vi "SUMMER SUNDAY BYTE[3].vi"() -> ()   [LabVIEW 2009]
uses:
  <vilib>/ULx/Create Channel.llb/ULx Create Channel (AI-Voltage-Basic).vi
  <vilib>/ULx/Read.llb/ULx Read (Analog DBL 1Chan 1Samp).vi
panel:
  out "POWER":bool
  out "data":dbl format="%_6g"
  out "xray":bool caption="BitValue"
  out "ENERGY LEVEL":dbl(knob) scale=0.0..15.0
  out "Beam Pot":dbl format="%_6g"
  out "READY 2":bool
  out "DUMP":bool
  out "POWER":bool
  out "?":bool
  out "?":bool
  out "?":bool
  out "?":bool
  out "?":bool
  out "?":bool
  out "?":bool
  out "?":bool
  out "?":bool
  out "?":bool
  out "OPEN":bool
  out "CLOSED":bool
  out "READY":bool
  out "FAULT":bool
  out "MAGNET FORCE":dbl(slide) scale=0.0..10.0
  out "READY":bool
  out "TEMPERATURE":dbl(slide) scale=0.0..100.0
  in  "stop":bool
  out "?":bool
  out "?":bool
  out "?":bool
  out "?":bool
  out "FAULT":bool
  out "POWER":bool
  out "FLOW IN GPM":dbl(knob) scale=0.0..15.0
  # "USERS LAB AREA"
  # "BEAM STATUS"
  # "ROOM"
  # "XRAY"
  # "PUMP STATION"
  # "MAGNET STATUS"
  # "ORBIT"
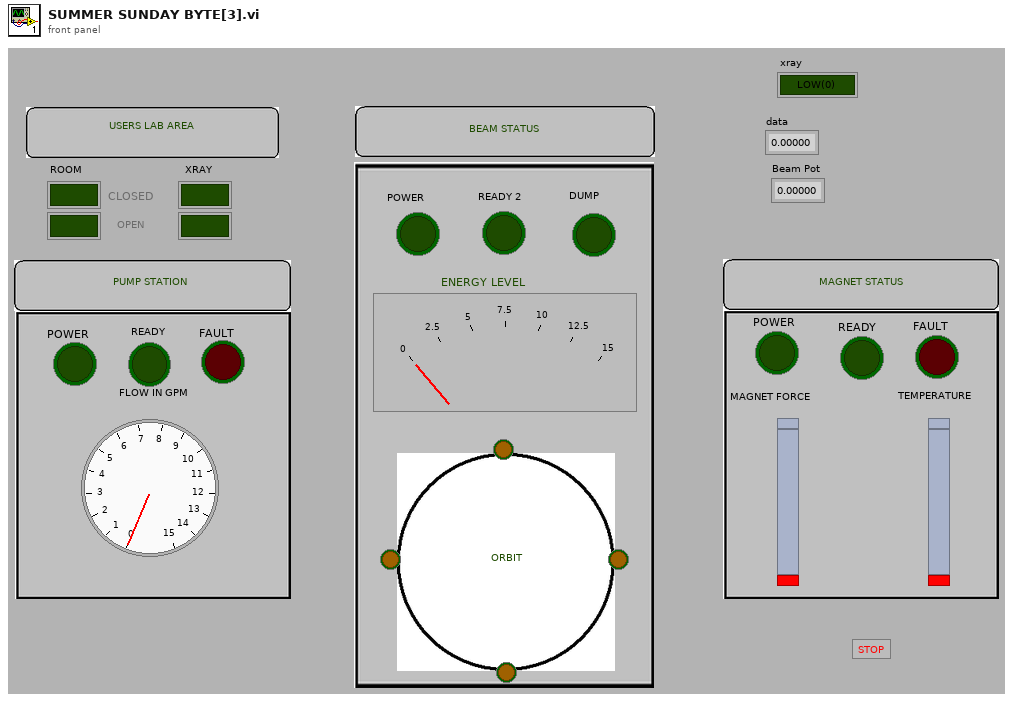
[diagram p1: front panel]
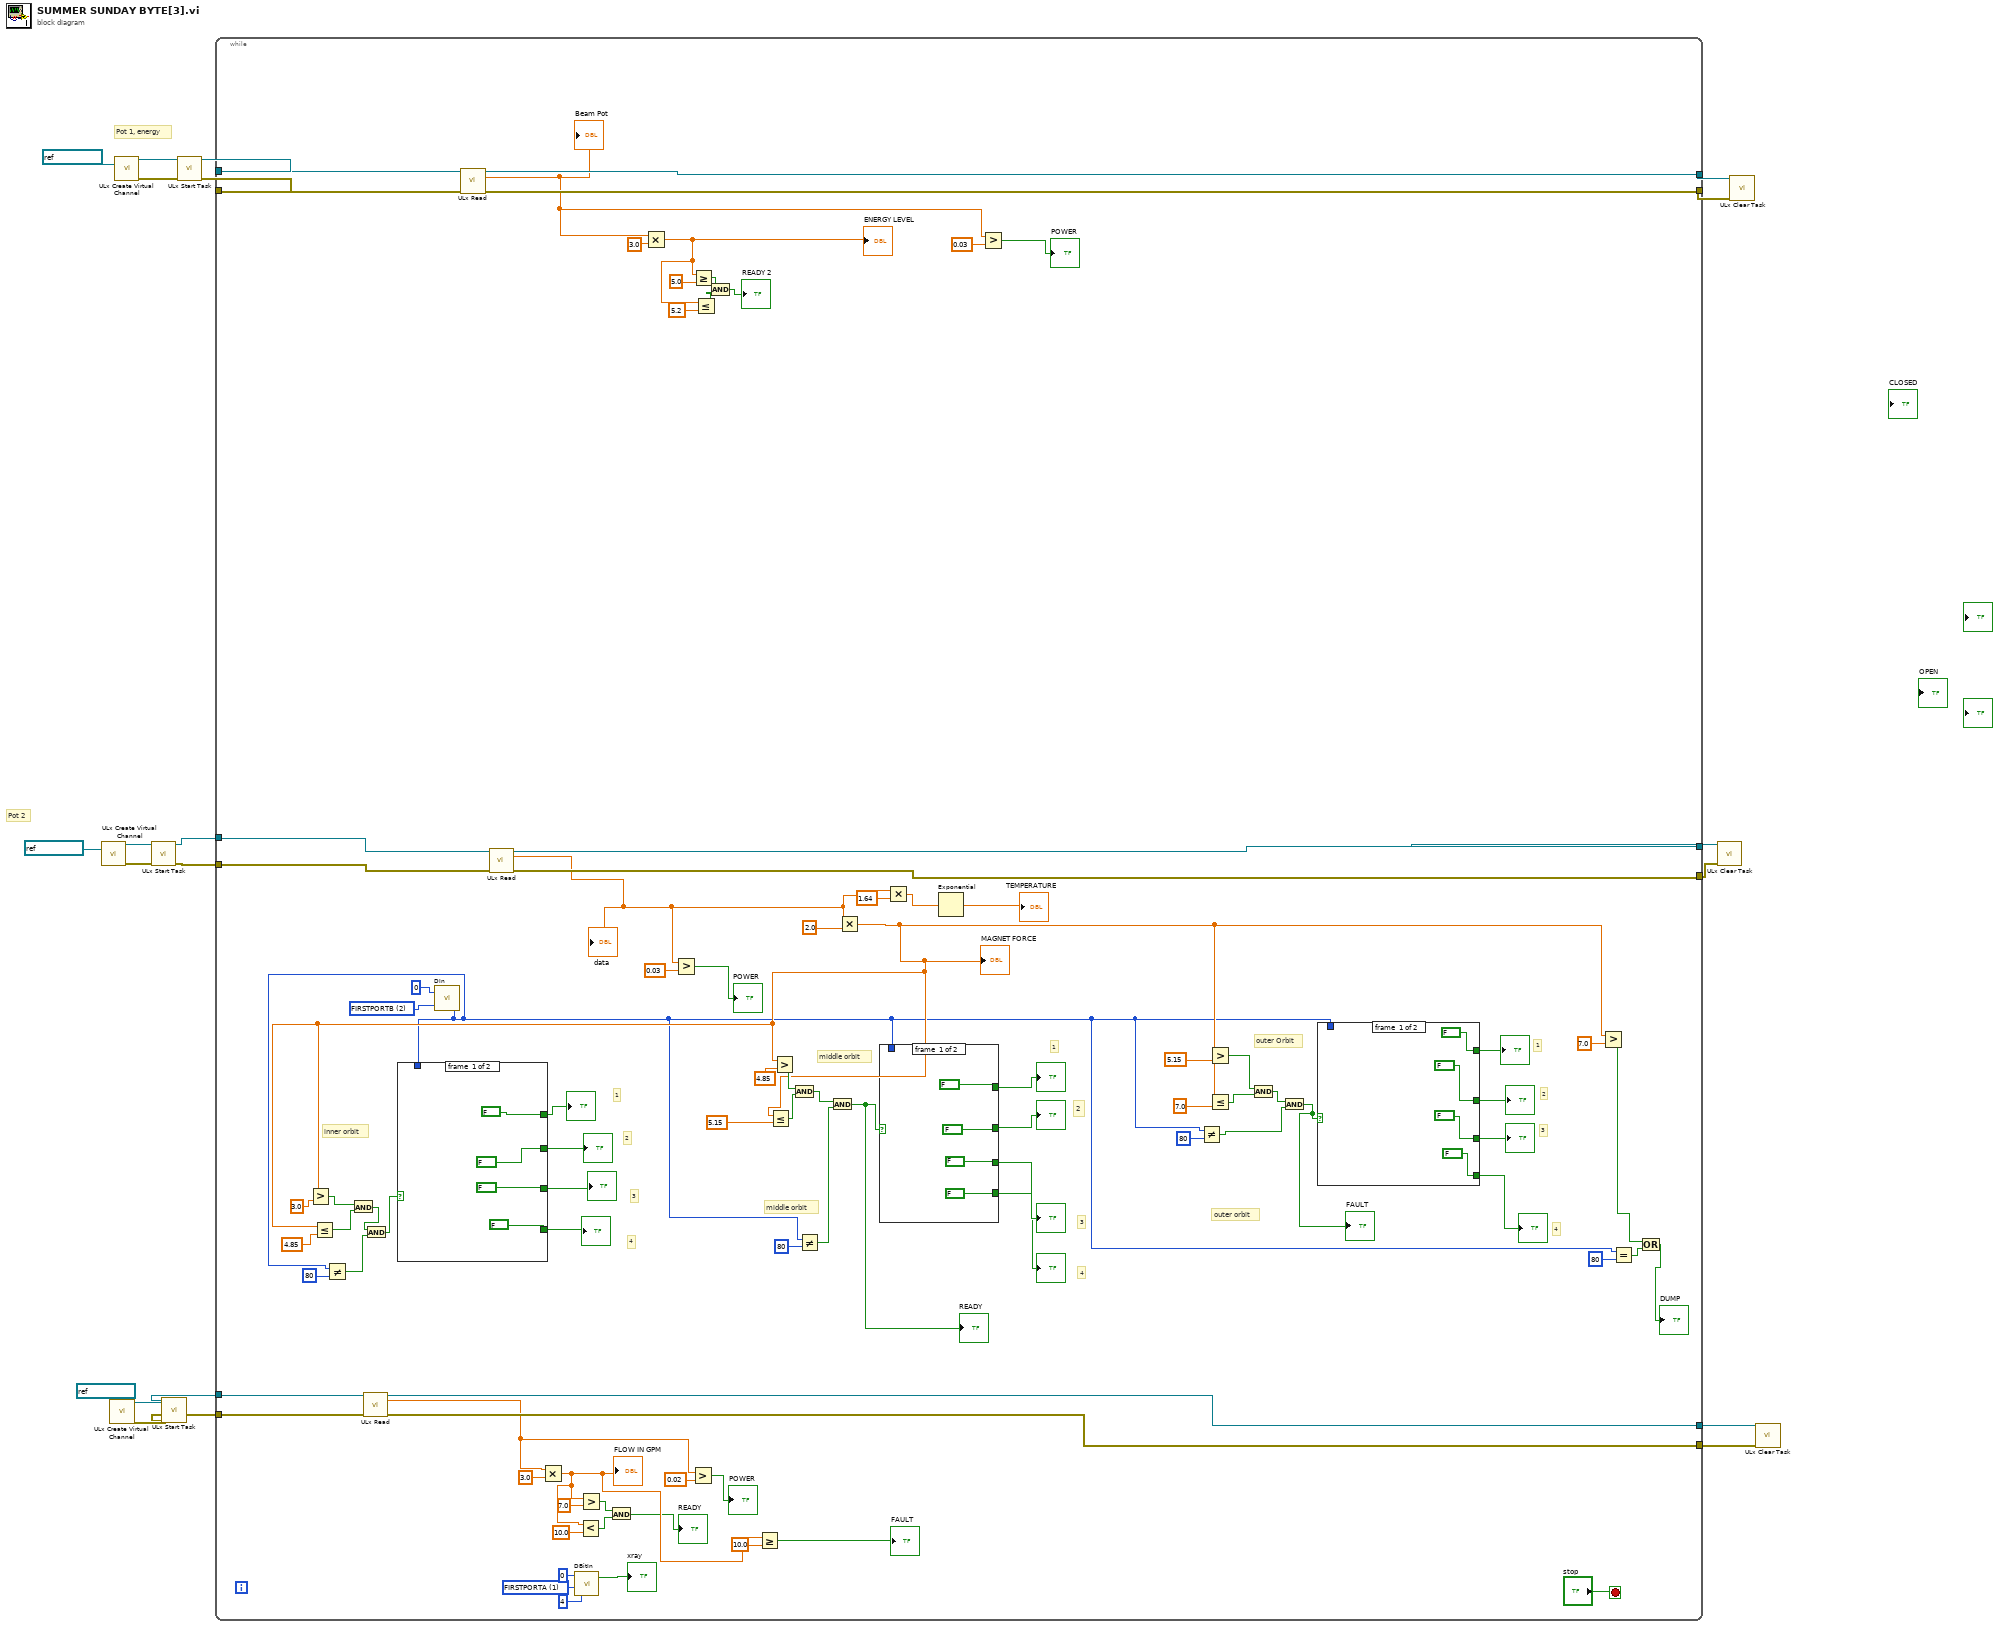
[diagram p0: block diagram]
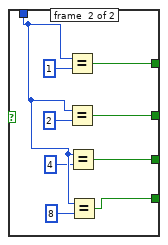
[diagram p2: hidden frame]
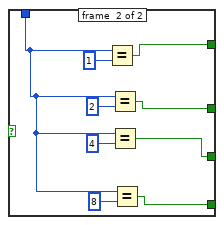
[diagram p3: hidden frame]
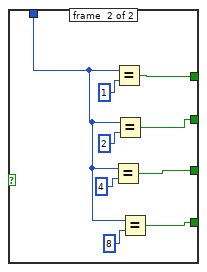
[diagram p4: hidden frame]
diagram:
  # "Pot 2"
  # "Pot 1, energy"
  n1 = call-poly <vilib>:"ULx Create Virtual Channel.vi"("physical channels"=refnum<k21> "Dev0/Ai1") -> ("task out"=w15:refnum<k24>, "error out"=w14:errorcluster)  [unwired: 13 in]
  n2 = call-poly <vilib>:"ULx Create Virtual Channel.vi"("physical channels"=refnum<k21> "Dev0/Ai2") -> ("task out"=w7:refnum<k24>, "error out"=w6:errorcluster)  [unwired: 13 in]
  n3 = call-poly <vilib>:"ULx Create Virtual Channel.vi"("physical channels"=refnum<k21> "Dev0/Ai0") -> ("task out"=w21:refnum<k24>, "error out"=w20:errorcluster)  [unwired: 13 in]
  n4 = call <vilib>:"ULx Start Task.vi"("task in"=w15, "error in"=w14) -> ("task out"=w13:refnum<k24>, "error out"=w12:errorcluster)  [unwired: 12 in]
  n5 = call <vilib>:"ULx Start Task.vi"("task in"=w7, "error in"=w6) -> ("task out"=w5:refnum<k24>, "error out"=w4:errorcluster)  [unwired: 12 in]
  n6 = call <vilib>:"ULx Start Task.vi"("task in"=w21, "error in"=w20) -> ("task out"=w19:refnum<k24>, "error out"=w18:errorcluster)  [unwired: 12 in]
  n7 = while {
    tunnel: w19 -> [w111]
    tunnel: w18 -> [w110]
    tunnel: [w109] -> w17
    tunnel: [w108] -> w16
    tunnel: w13 -> [w106]
    tunnel: w12 -> [w105]
    tunnel: [w104] -> w11
    tunnel: [w103] -> w10
    tunnel: w5 -> [w61]
    tunnel: w4 -> [w60]
    tunnel: [w59] -> w2
    tunnel: [w58] -> w1
    stop <- "stop" stop-if-true
    w56 = 1 items=["AUXPORT", "FIRSTPORTA"] ("PortType")
    w80 = 2 items=["AUXPORT", "FIRSTPORTA", "FIRSTPORTB", "FIRSTPORTCL", "FIRSTPORTCH", "SECONDPORTA", "SECONDPORTB", "SECONDPORTCL", "SECONDPORTCH", "THIRDPORTA", "THIRDPORTB", "THIRDPORTCL", "THIRDPORTCH", "FOURTHPORTA", "FOURTHPORTB", "FOURTHPORTCL", "FOURTHPORTCH", "FIFTHPORTA", "FIFTHPORTB", "FIFTHPORTCL", "FIFTHPORTCH", "SIXTHPORTA", "SIXTHPORTB", "SIXTHPORTCL", "SIXTHPORTCH", "SEVENTHPORTA", "SEVENTHPORTB", "SEVENTHPORTCL", "SEVENTHPORTCH", "EIGTHPORTA", "EIGHTHPORTB", "EIGHTHPORTCL", "EIGHTHPORTCH"] ("PortNum")
    # "outer Orbit"
    # "middle orbit"
    # "4"
    # "3"
    # "2"
    # "1"
    # "1"
    # "2"
    # "3"
    # "4"
    # "4"
    # "3"
    # "2"
    # "1"
    # "outer orbit"
    # "inner orbit"
    # "middle orbit"
    n8 = call-poly <vilib>:"ULx Read.vi"("task in"=w61, "error in"=w60) -> ("task out"=w59:refnum<k24>, "data"=w48:dbl, "error out"=w58:errorcluster)  [unwired: 11 in]
    n9 = call <menus>:"DIn.VI"("PortNum"=w80, "BoardNum"=u32 0) -> ("DataValue"=w68:i16)  [unwired: 1 out]
    n10 = Not Equal?(x=w68, y=i16 80) -> (x != y?=w90:bool)
    n11 = call-poly <vilib>:"ULx Read.vi"("task in"=w111, "error in"=w110) -> ("task out"=w109:refnum<k24>, "data"=w22:dbl, "error out"=w108:errorcluster)  [unwired: 11 in]
    "Beam Pot" <- w22
    n12 = call-poly <vilib>:"ULx Read.vi"("task in"=w106, "error in"=w105) -> ("task out"=w104:refnum<k24>, "data"=w26:dbl, "error out"=w103:errorcluster)  [unwired: 11 in]
    "data" <- w26
    n13 = Multiply(x=w48, y=3.0) -> (x*y=w33:dbl)
    "FLOW IN GPM" <- w33
    n14 = call <menus>:"DBitIn.VI"("BitNum"=4, "PortType"=w56, "BoardNum"=u32 0) -> ("BitValue"=→"xray":bool)  [unwired: 1 out]
    n15 = Less?(x=w33, y=10.0) -> (x < y?=w31:bool)
    n16 = Greater?(x=w33, y=7.0) -> (0:w32:bool)
    n17 = And(x=w32, y=w31) -> (x .and. y?=→"READY":bool)
    n18 = Multiply(x=w22, y=3.0) -> (x*y=w43:dbl)
    "ENERGY LEVEL" <- w43
    n19 = Greater?(x=w26, y=0.03) -> (0:→"POWER":bool)
    n20 = Greater?(x=w48, y=0.02) -> (0:→"POWER":bool)
    n21 = Greater Or Equal?(x=w43, y=5.0) -> (x >= y?=w40:bool)
    n22 = Less Or Equal?(x=w43, y=5.2) -> (x <= y?=w39:bool)
    n23 = And(x=w40, y=w39) -> (x .and. y?=→"READY 2":bool)
    n24 = Greater Or Equal?(x=w33, y=10.0) -> (x >= y?=→"FAULT":bool)
    n25 = Not Equal?(x=w68, y=i16 80) -> (x != y?=w76:bool)
    n26 = Multiply(x=w26, y=2.0) -> (x*y=w83:dbl)
    "MAGNET FORCE" <- w83
    n27 = Greater?(x=w83, y=3.0) -> (0:w99:bool)
    n28 = Less Or Equal?(x=w83, y=4.85) -> (x <= y?=w100:bool)
    n29 = And(x=w99, y=w100) -> (x .and. y?=w92:bool)
    n30 = And(x=w92, y=w90) -> (x .and. y?=w91:bool)
    n31 = case shown="True" w91 {
      tunnel: [FALSE w146] -> w64
      tunnel: [FALSE w145] -> w65
      tunnel: [FALSE w144] -> w62
      tunnel: [FALSE w143] -> w63
      tunnel: w68 -> [_ w151]
      frame #0 {
      }
      frame #1 {
        n32 = Equal?(x=w151, y=i16 4) -> (x = y?=w144:bool)
        n33 = Equal?(x=w151, y=i16 1) -> (x = y?=w146:bool)
        n34 = Equal?(x=w151, y=i16 2) -> (x = y?=w145:bool)
        n35 = Equal?(x=w151, y=i16 8) -> (x = y?=w143:bool)
      }
    }
    "?" <- w65
    "?" <- w62
    "?" <- w63
    "?" <- w64
    n36 = Less Or Equal?(x=w83, y=5.15) -> (x <= y?=w96:bool)
    n37 = Greater?(x=w83, y=4.85) -> (0:w97:bool)
    n38 = And(x=w97, y=w96) -> (x .and. y?=w89:bool)
    n39 = And(x=w89, y=w76) -> (x .and. y?=w46:bool)
    "READY" <- w46
    n40 = case shown="True" w46 {
      tunnel: [FALSE w125] -> w75
      tunnel: [FALSE w124] -> w74
      tunnel: [FALSE w123] -> w73
      tunnel: [FALSE w122] -> w72
      tunnel: w68 -> [_ w121]
      frame #0 {
      }
      frame #1 {
        n41 = Equal?(x=w121, y=i16 1) -> (x = y?=w125:bool)
        n42 = Equal?(x=w121, y=i16 2) -> (x = y?=w124:bool)
        n43 = Equal?(x=w121, y=i16 4) -> (x = y?=w123:bool)
        n44 = Equal?(x=w121, y=i16 8) -> (x = y?=w122:bool)
      }
    }
    "?" <- w75
    "?" <- w74
    "?" <- w73
    "?" <- w72
    n45 = Multiply(x=w26, y=1.64) -> (x*y=w24:dbl)
    n46 = Exponential(1:w24) -> (0:→"TEMPERATURE":dbl)
    n47 = Greater?(x=w22, y=0.03) -> (0:→"POWER":bool)
    n48 = Not Equal?(x=w68, y=i16 80) -> (x != y?=w70:bool)
    n49 = Greater?(x=w83, y=5.15) -> (0:w94:bool)
    n50 = Less Or Equal?(x=w83, y=7.0) -> (x <= y?=w93:bool)
    n51 = And(x=w94, y=w93) -> (x .and. y?=w82:bool)
    n52 = And(x=w82, y=w70) -> (x .and. y?=w27:bool)
    "FAULT" <- w27
    n53 = case shown="True" w27 {
      tunnel: [FALSE w130] -> w87
      tunnel: [FALSE w131] -> w86
      tunnel: [FALSE w132] -> w85
      tunnel: [FALSE w133] -> w84
      tunnel: w68 -> [_ w138]
      frame #0 {
      }
      frame #1 {
        n54 = Equal?(x=w138, y=i16 1) -> (x = y?=w133:bool)
        n55 = Equal?(x=w138, y=i16 2) -> (x = y?=w132:bool)
        n56 = Equal?(x=w138, y=i16 4) -> (x = y?=w131:bool)
        n57 = Equal?(x=w138, y=i16 8) -> (x = y?=w130:bool)
      }
    }
    "?" <- w84
    "?" <- w85
    "?" <- w86
    "?" <- w87
    n58 = Greater?(x=w83, y=7.0) -> (0:w28:bool)
    n59 = Equal?(x=w68, y=i16 80) -> (x = y?=w66:bool)
    n60 = Or(x=w28, y=w66) -> (x .or. y?=→"DUMP":bool)
  }
  n61 = call <vilib>:"ULx Clear Task.vi"("task in"=w11, "error in"=w10) -> ()  [unwired: 13 in, 1 out]
  n62 = call <vilib>:"ULx Clear Task.vi"("task in"=w17, "error in"=w16) -> ()  [unwired: 13 in, 1 out]
  n63 = call <vilib>:"ULx Clear Task.vi"("task in"=w2, "error in"=w1) -> ()  [unwired: 13 in, 1 out]
